vi "Wait on Listener.vi"(8 "error in (no error)":errorcluster, 9 "timeout ms (5000)":i32=5000, 11 "Socket Listener in":refnum<class "Socket Listener.lvclass">) -> (0 "error out":errorcluster, 2 "Socket out":refnum<class "Socket.lvclass">, 3 "Socket Listener out":refnum<class "Socket Listener.lvclass">)   [LabVIEW 2013, in "Sockets.lvlib" / "Socket Listener.lvclass"]
doc: "Listens for an incoming TCP socket connection on the given port."
uses:
  Socket Listener.lvclass
  Socket/Socket.lvclass
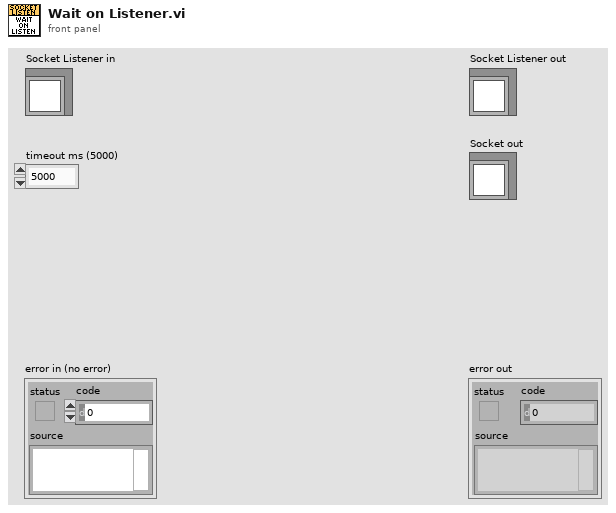
[diagram p1: front panel]
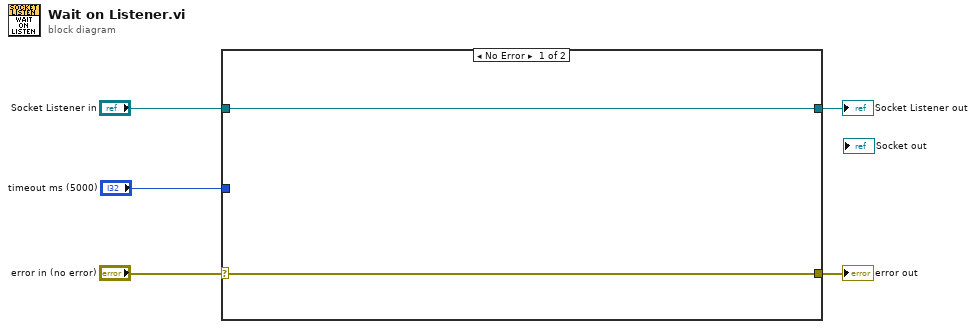
[diagram p0: block diagram]
diagram:
  n1 = case shown="No Error" "error in (no error)" {
    selector: "error in (no error)" -> [w6 w9]
    tunnel: [w6 w9] -> w4
    tunnel: [w7 w8] -> w2
    tunnel: "Socket Listener in" -> [w7 w8]
    tunnel: "timeout ms (5000)" -> [_ _]
    frame No Error {
    }
    frame Error {
    }
  }
  "error out" <- w4
  "Socket Listener out" <- w2
